vi "Keyence.Cmd.ParametersBank.Set.vi"(6 "Timeout [ms] (1000)":i32=1000, 7 "Bank":i32, 8 "error in":errorcluster, 9 "Parameters":string, 10 "Cmd":T1, 11 "cID in":refnum<k5>) -> (0 "error out":errorcluster, 1 "OK?":bool, 2 "Response":string, 3 "cID out":refnum<k5>)   [LabVIEW 2015]
uses:
  Keyence.Cmd.ParametersBank.ctl
panel:
  out "response 2":string
  out "response 1":string
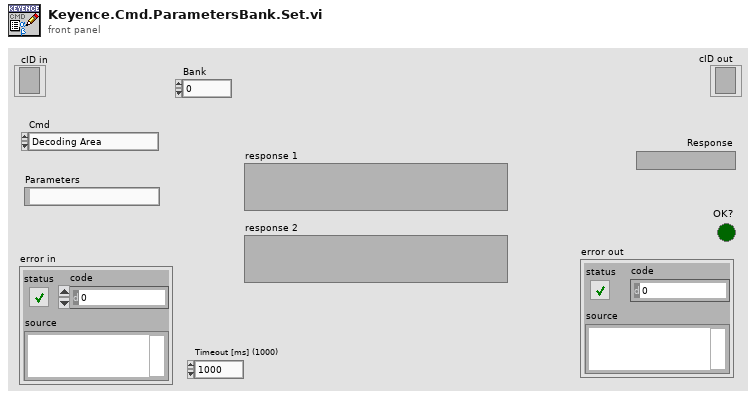
[diagram p1: front panel]
types:
  T1 = typedef "Keyence.Cmd.ParametersBank.ctl" = enum16{"Decoding Area", "Scan.DynamicRange"}
  T2 = enum16{"Standard", "Buffered", "CRLF", "Immediate"}
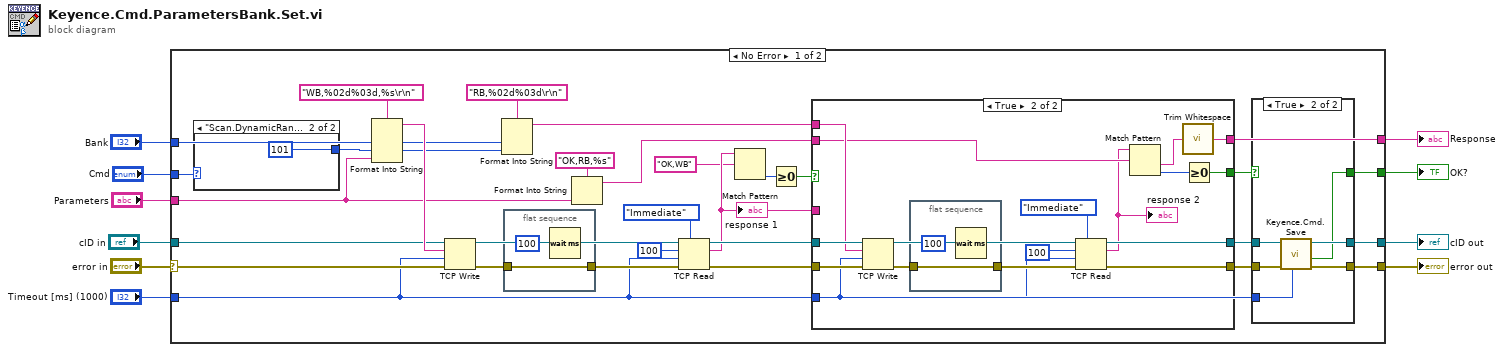
[diagram p0: block diagram]
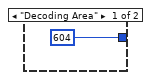
[diagram p2: hidden frame]
diagram:
  n1 = case shown="No Error" "error in" {
    selector: "error in" -> [w28 w77]
    tunnel: "Timeout [ms] (1000)" -> [w12 _]
    tunnel: "Cmd" -> [w39 _]
    tunnel: "Bank" -> [w32 _]
    tunnel: "Parameters" -> [w20 _]
    tunnel: "cID in" -> [w29 w78]
    tunnel: [w15 w78] -> w5
    tunnel: [w16 w77] -> w2
    tunnel: [w19 _] -> w4
    tunnel: [w13 _] -> w3
    frame No Error {
      n2 = case shown="\"Scan.DynamicRange\"" w39 {
        tunnel: [604 101] -> w31
        frame "Decoding Area" {
        }
        frame "Scan.DynamicRange" {
        }
      }
      n3 = Format Into String(format string="WB,%02d%03d,%s\r\n", w32, w31, w20) -> (resulting string=w38:string)  [unwired: 2 in, 1 out]
      n4 = TCP Write(connection ID=w29, data in=w38, error in (no error)=w28, 9:w12) -> (connection ID out=w36:refnum<k5>, error out=w41:errorcluster)  [unwired: 1 out]
      n5 = Format Into String(format string="RB,%02d%03d\r\n", w32, w31) -> (resulting string=w26:string)  [unwired: 2 in, 1 out]
      n6 = flat-sequence {
        tunnel: w41 -> [w43]
        tunnel: [w43] -> w37
        frame #0 {
          n7 = Wait (ms)(milliseconds to wait=u32 100) -> ()  [unwired: 1 out]
        }
      }
      n8 = Format Into String(format string="OK,RB,%s" ("regular expression"), w20) -> (resulting string=w11:string)  [unwired: 2 in, 1 out]
      n9 = TCP Read(connection ID=w36, bytes to read=100, error in (no error)=w37, 7:T2."Immediate" ("mode (standard)"), 9:w12) -> (connection ID out=w34:refnum<k5>, data out=w30:string, error out=w35:errorcluster)
      "response 1" <- w30
      n10 = Match Pattern(string=w30, regular expression="OK,WB") -> (offset past match=w22:i32)  [unwired: 1 in, 3 out]
      n11 = Greater Or Equal To 0?(x=w22) -> (x >= 0?=w33:bool)
      n12 = case shown="True" w33 {
        tunnel: w35 -> [w47 w65]
        tunnel: w34 -> [w48 w64]
        tunnel: [w48 w54] -> w17
        tunnel: [w47 w55] -> w18
        tunnel: w12 -> [_ w57]
        tunnel: [_ w53] -> w14
        tunnel: [w46 w49] -> w19
        tunnel: w30 -> [w46 _]
        tunnel: w26 -> [_ w63]
        tunnel: w11 -> [_ w52]
        frame False {
        }
        frame True {
          n13 = TCP Write(connection ID=w64, data in=w63, error in (no error)=w65, 9:w57) -> (connection ID out=w56:refnum<k5>, error out=w59:errorcluster)  [unwired: 1 out]
          n14 = flat-sequence {
            tunnel: w59 -> [w67]
            tunnel: [w67] -> w58
            frame #0 {
              n15 = Wait (ms)(milliseconds to wait=u32 100) -> ()  [unwired: 1 out]
            }
          }
          n16 = TCP Read(connection ID=w56, bytes to read=100, error in (no error)=w58, 7:T2."Immediate" ("mode (standard)"), 9:w57) -> (connection ID out=w54:refnum<k5>, data out=w51:string, error out=w55:errorcluster)
          "response 2" <- w51
          n17 = Match Pattern(string=w51, regular expression=w52) -> (after substring=w50:string, offset past match=w62:i32)  [unwired: 1 in, 2 out]
          n18 = call <vilib>:"Trim Whitespace.vi"("string"=w50) -> ("trimmed string"=w49:string)  [unwired: 1 in]
          n19 = Greater Or Equal To 0?(x=w62) -> (x >= 0?=w53:bool)
        }
      }
      n20 = case shown="True" w14 {
        selector: w14 -> [w68 _]
        tunnel: [w70 w76] -> w15
        tunnel: [w69 w75] -> w16
        tunnel: w18 -> [w69 w74]
        tunnel: w17 -> [w70 w73]
        tunnel: w12 -> [_ w72]
        tunnel: [w68 w71] -> w13
        frame False {
        }
        frame True {
          n21 = call "Keyence.Cmd.Save.vi"("Timeout [ms] (1000)"=w72, "error in"=w74, "cID in"=w73) -> ("error out"=w75:errorcluster, "OK?"=w71:bool, "cID out"=w76:refnum<k5>)  [unwired: 6 in]
        }
      }
    }
    frame Error {
    }
  }
  "cID out" <- w5
  "Response" <- w4
  "OK?" <- w3
  "error out" <- w2
